vi "Reset Timer.vi"(8 "error in (no error)":errorcluster, 11 "timer":T1) -> (0 "error out":errorcluster, 3 "timer out":T1)   [LabVIEW 2011]
doc: "Resets the timer.\n\n© Copyright 1999\nCal-Bay Systems, Inc.\nwritten by James Kring"
uses:
  Timer Refnum.ctl
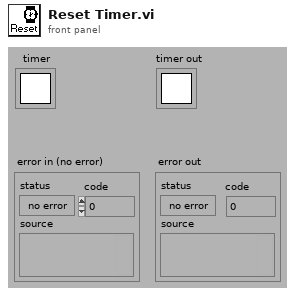
[diagram p1: front panel]
types:
  T1 = typedef "Timer Refnum.ctl" = refnum<k1>
  T2 = enum16{"open ref", "lookup ref", "close ref", "test ref", "start", "stop", "wait", "reset", "increment # waiting", "decrement #waiting"}
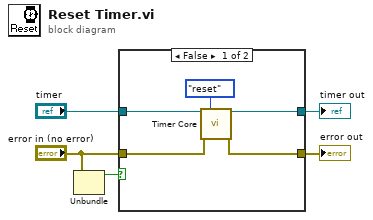
[diagram p0: block diagram]
diagram:
  n1 = Unbundle("error in (no error)") -> ("status"=w3:bool)  [unwired: 2 out]
  n2 = case shown="False" w3 {
    tunnel: "timer" -> [w10 w11]
    tunnel: [w9 w11] -> w4
    tunnel: "error in (no error)" -> [w7 w12]
    tunnel: [w8 w12] -> w1
    frame False {
      n3 = call "Timer Core.vi"("timer"=w10, "function"=T2."reset", "error in (no error)"=w7) -> ("timer out"=w9:T1, "error out"=w8:errorcluster)  [unwired: 6 in, 5 out]
    }
    frame True {
    }
  }
  "timer out" <- w4
  "error out" <- w1
